vi "TrianglesSubtract.vi"(10 "Point3D":T1, 11 "TrianglesIn":T2[](array[typedef])) -> (3 "TrianglesOut":T2[](array[typedef]))   [LabVIEW 2014]
uses:
  TypeDefs/TriangleFace.ctl
  TypeDefs/Point3D.ctl
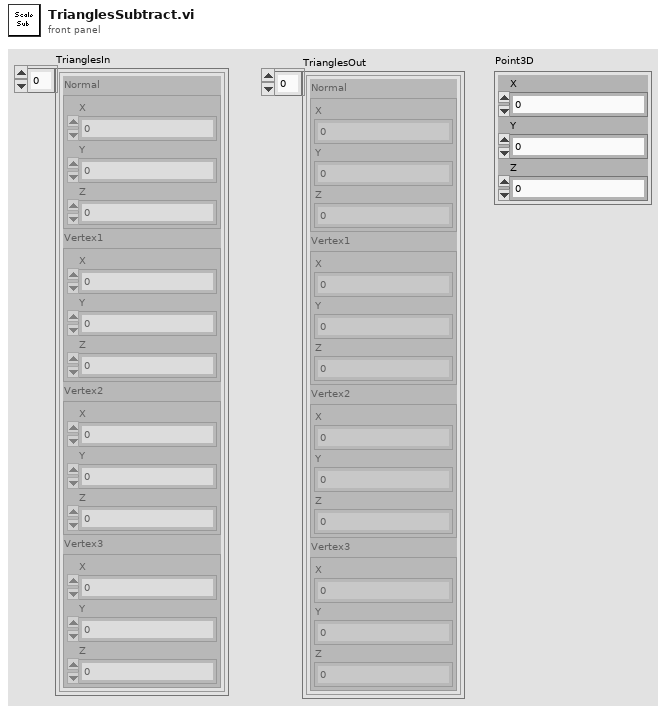
[diagram p1: front panel]
types:
  T1 = typedef "Point3D.ctl" = cluster{"X":sgl, "Y":sgl, "Z":sgl}
  T2 = typedef "TriangleFace.ctl" = cluster{"Normal":T1, "Vertex1":T1, "Vertex2":T1, "Vertex3":T1}
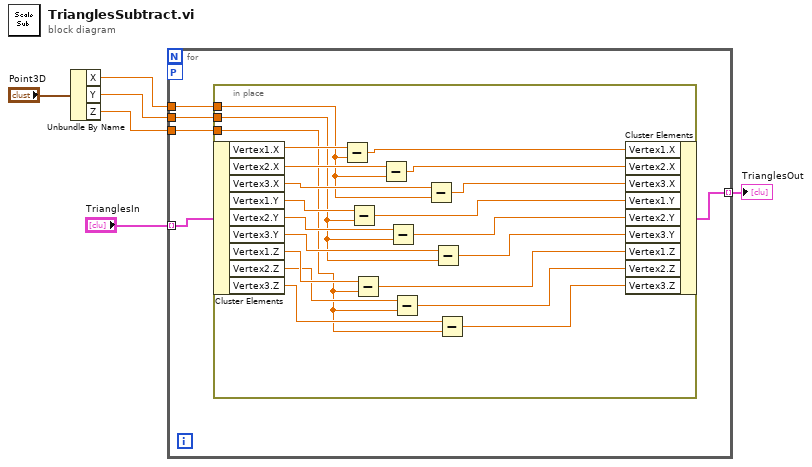
[diagram p0: block diagram]
diagram:
  n1 = Unbundle By Name("Point3D") -> ("X"=w3:sgl, "Y"=w2:sgl, "Z"=w1:sgl)
  n2 = for {
    tunnel: "TrianglesIn" -> [w11] mode=indexing
    tunnel: w3 -> [w10]
    tunnel: [w9] -> w5 mode=indexing
    tunnel: w2 -> [w8]
    tunnel: w1 -> [w7]
    workers-P: _ -> [_]
    n3 = in-place {
      in-place-border: w10 -> [w17]
      in-place-border: w8 -> [w13]
      in-place-border: w7 -> [w12]
      n4 = in-place-cluster #1(w11) -> ("Vertex1.X"=w32:sgl, "Vertex2.X"=w31:sgl, "Vertex3.X"=w29:sgl, "Vertex1.Y"=w26:sgl, "Vertex2.Y"=w25:sgl, "Vertex3.Y"=w24:sgl, "Vertex1.Z"=w20:sgl, "Vertex2.Z"=w19:sgl, "Vertex3.Z"=w18:sgl)
      n5 = Subtract(x=w32, y=w17) -> (x-y=w27:sgl)
      n6 = Subtract(x=w26, y=w13) -> (x-y=w23:sgl)
      n7 = Subtract(x=w20, y=w12) -> (x-y=w16:sgl)
      n8 = Subtract(x=w31, y=w17) -> (x-y=w30:sgl)
      n9 = Subtract(x=w25, y=w13) -> (x-y=w22:sgl)
      n10 = Subtract(x=w19, y=w12) -> (x-y=w15:sgl)
      n11 = Subtract(x=w29, y=w17) -> (x-y=w28:sgl)
      n12 = Subtract(x=w24, y=w13) -> (x-y=w21:sgl)
      n13 = Subtract(x=w18, y=w12) -> (x-y=w14:sgl)
      n14 = in-place-cluster #1("Vertex1.X"=w27, "Vertex2.X"=w30, "Vertex3.X"=w28, "Vertex1.Y"=w23, "Vertex2.Y"=w22, "Vertex3.Y"=w21, "Vertex1.Z"=w16, "Vertex2.Z"=w15, "Vertex3.Z"=w14) -> (w9:T2)
    }
  }
  "TrianglesOut" <- w5
